vi "Poll iRobot and Accelerometer.vi"(8 "error in":errorcluster, 11 "UART port in":T10) -> (0 "error out":errorcluster, 1 "Acceleration (g)":T1 {"z axis (g)" format="%.3f"; "y axis (g)" format="%.3f"; "x axis (g)" format="%.3f"}, 2 "iRobot SensorGroup6":T2={"Bumps + Wheel Drops"={"Wheeldrop Caster"=FALSE, "Wheeldrop Left"=FALSE, "Wheeldrop Right"=FALSE, "Bump Left"=FALSE, "Bump Right"=FALSE}, "Wall"=FALSE, "Cliff Left"=FALSE, "Cliff Front Left"=FALSE, "Cliff Front Right"=FALSE, "Cliff Right"=FALSE, "Wall Signal"=0, "Cliff Left Signal"=0, "Cliff Front Left Signal"=0, "Cliff Front Right Signal"=0, "Cliff Right Signal"=0, "Buttons"={"Advance"=FALSE, "Play"=FALSE}, "Virtual Wall"=FALSE, "# Stream Packets"=0, "Requested Velocity (mm/s)"=0, "Requested Radius (mm)"=0, "Requested Right Wheel Velocity (mm/s)"=0, "Requested Left Wheel Velocity (mm/s)"=0, "Distance (mm)"=0, "Angle (deg)"=0, "Song Playing"=FALSE, "Song Number"=0, "Charging State"=enum."Not Charging", "Voltage (mV)"=0, "Current (mA)"=0, "Battery Temperature (deg C)"=0, "Battery Charge (mAh)"=0, "Battery Capacity (mAh)"=0, "Charging Sources"={"Internal Charger"=FALSE, "Home Base"=FALSE}, "OI Mode"=enum."Off", "Digital Inputs"={"Digital Input 0"=FALSE, "Digital Input 1"=FALSE, "Digital Input 2"=FALSE, "Digital Input 3"=FALSE, "Device Detect"=FALSE}, "Drivers & Wheel Overcurrent"={"Low-Side Driver 0"=FALSE, "Low-Side Driver 1"=FALSE, "Low-Side Driver 2"=FALSE, "Left Wheel"=FALSE, "Right Wheel"=FALSE}, "Analog Signal"=0, "Infrared"=255} {"Infrared" format="%02x"}, 3 "UART port out":T10, 5 "net angle (deg)":i32, 7 "net distance (mm)":i32)   [LabVIEW 2013]
uses:
  iRobot/Advanced/UART/iRobot UART Port Type.ctl
  iRobot/Sensor/Sensor Group 6.ctl
  iRobot/Sensor/Bumps + Wheel Drops.ctl
  iRobot/Sensor/Buttons.ctl
  iRobot/Sensor/Charging State.ctl
  iRobot/Sensor/Charging Sources Available.ctl
  iRobot/Sensor/OI Mode.ctl
  iRobot/Sensor/Cargo Bay Digital Inputs.ctl
  iRobot/Sensor/Low-Side Driver + Wheel Overcurrent.ctl
  iRobot/Sensor/Accelerometer.ctl
panel:
  # "Electrical: charging, battery, OI mode"
  # "Sensors: bump, cliff, button, wheel drop, wall, virtual wall"
  # "Motion: distance, angle, requested velocity"
  # "Cargo Bay: I/O, overcurrent, infrared"
  # "Song"
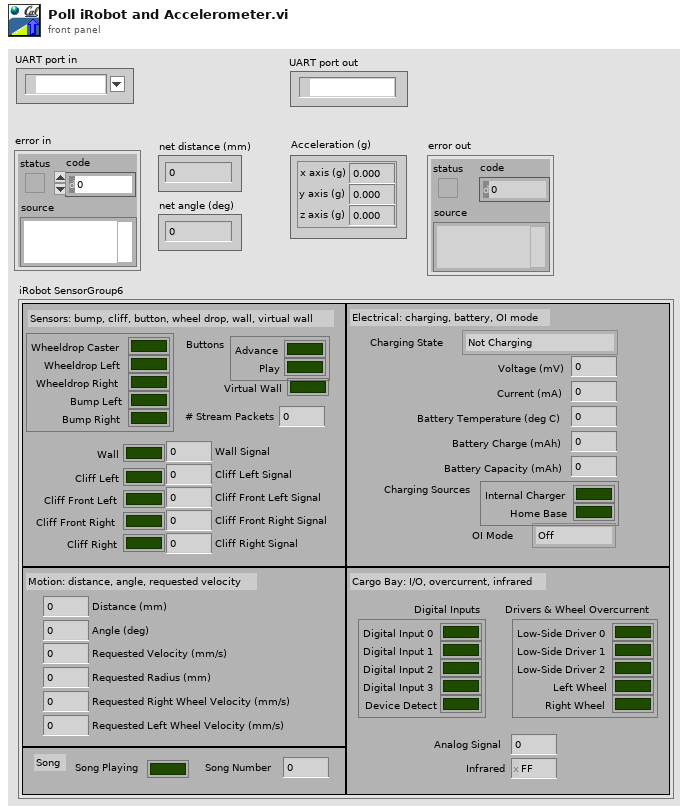
[diagram p1: front panel]
types:
  T1 = typedef "Accelerometer.ctl" = cluster{"x axis (g)":dbl, "y axis (g)":dbl, "z axis (g)":dbl}
  T2 = typedef "Sensor Group 6.ctl" = cluster{"Bumps + Wheel Drops":T3, "Wall":bool, "Cliff Left":bool, "Cliff Front Left":bool, "Cliff Front Right":bool, "Cliff Right":bool, "Wall Signal":u16, "Cliff Left Signal":u16, "Cliff Front Left Signal":u16, "Cliff Front Right Signal":u16, "Cliff Right Signal":u16, "Buttons":T4, "Virtual Wall":bool, "# Stream Packets":u8, "Requested Velocity (mm/s)":i16, "Requested Radius (mm)":i16, "Requested Right Wheel Velocity (mm/s)":i16, "Requested Left Wheel Velocity (mm/s)":i16, "Distance (mm)":i32, "Angle (deg)":i32, "Song Playing":bool, "Song Number":u8, "Charging State":T5, "Voltage (mV)":u16, "Current (mA)":i16, "Battery Temperature (deg C)":i8, "Battery Charge (mAh)":u16, "Battery Capacity (mAh)":u16, "Charging Sources":T6, "OI Mode":T7, "Digital Inputs":T8, "Drivers & Wheel Overcurrent":T9, "Analog Signal":u16, "Infrared":u8}
  T3 = typedef "Bumps + Wheel Drops.ctl" = cluster{"Wheeldrop Caster":bool, "Wheeldrop Left":bool, "Wheeldrop Right":bool, "Bump Left":bool, "Bump Right":bool}
  T4 = typedef "Buttons.ctl" = cluster{"Advance":bool, "Play":bool}
  T5 = typedef "Charging State.ctl" = enum16{"Not Charging", "Reconditioning Charging", "Full Charging", "Trickle Charging", "Waiting", "Charging Fault Condition"}
  T6 = typedef "Charging Sources Available.ctl" = cluster{"Internal Charger":bool, "Home Base":bool}
  T7 = typedef "OI Mode.ctl" = enum16{"Off", "Passive", "Safe", "Full"}
  T8 = typedef "Cargo Bay Digital Inputs.ctl" = cluster{"Digital Input 0":bool, "Digital Input 1":bool, "Digital Input 2":bool, "Digital Input 3":bool, "Device Detect":bool}
  T9 = typedef "Low-Side Driver + Wheel Overcurrent.ctl" = cluster{"Low-Side Driver 0":bool, "Low-Side Driver 1":bool, "Low-Side Driver 2":bool, "Left Wheel":bool, "Right Wheel":bool}
  T10 = typedef "iRobot UART Port Type.ctl" = refnum<visa-resource-name>
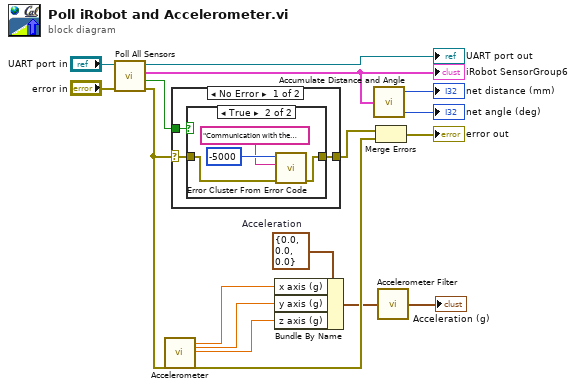
[diagram p0: block diagram]
diagram:
  w8 = T1 {"x axis (g)"=0.0, "y axis (g)"=0.0, "z axis (g)"=0.0}  # Acceleration
  n1 = call "Poll All Sensors.vi"("error in"="error in", "UART port in"="UART port in") -> ("error out"=w7:errorcluster, "Timed Out?"=w11:bool, "iRobot Sensors"=w17:T2, "UART port out"=→"UART port out":T10)  [unwired: 6 in]
  "iRobot SensorGroup6" <- w17
  n2 = call "Accelerometer"("error in (no error)"=w7) -> ("X-Axis"=w5:dbl, "Y-Axis"=w4:dbl, "Z-Axis"=w3:dbl, "error out"=w6:errorcluster)  [unwired: 23 in]
  n3 = case shown="No Error" w7 {
    selector: w7 -> [w18 w26]
    tunnel: w11 -> [w20 _]
    tunnel: [w19 w26] -> w9
    frame No Error {
      n4 = case shown="True" w20 {
        tunnel: [w21 w22] -> w19
        tunnel: w18 -> [w21 w25]
        frame False {
        }
        frame True {
          n5 = call <vilib>:"Error Cluster From Error Code.vi"("error in (no error)"=w25, "error message (\"\")"="Communication with the iRobot Create timed out." ("source"), "error code (0)"=-5000 ("code")) -> ("error out"=w22:errorcluster)  [unwired: 6 in]
        }
      }
    }
    frame Error {
    }
  }
  n6 = Bundle By Name(cluster=w8, "x axis (g)"=w5, "y axis (g)"=w4, "z axis (g)"=w3) -> (w2:T1)
  n7 = call "Accumulate Distance and Angle.vi"("iRobot SensorGroup6"=w17) -> ("net angle (mm)"=→"net angle (deg)":i32, "net distance (mm)"=→"net distance (mm)":i32)  [unwired: 3 in]
  n8 = Merge Errors(w9, w6) -> (→"error out":errorcluster)
  n9 = call "Accelerometer Filter.vi"("accelerometer (g)"=w2) -> ("filtered accelerometer (g)"=→"Acceleration (g)":T1)  [unwired: 3 in]
